vi "Activation Message Loop.vi"(8 "error in (no error)":errorcluster) -> (0 "error out":errorcluster)   [LabVIEW 2020, in "OPC.lvlib"]
doc: "Message loop for handling messages pertaining to the acquisition of data from the hardware."
uses:
  OPC.lvlib
  support/PCT FGV CMD.ctl
  Acquisition State.ctl
  AM Configuration.ctl
  support/Message Queue/Message Cluster.ctl
  support/Message Queue/Enqueue Message (Single).vi
  support/Message Queue/Message Queue.lvlib
  <vilib>/ErrorRing/Error Ring.xnode
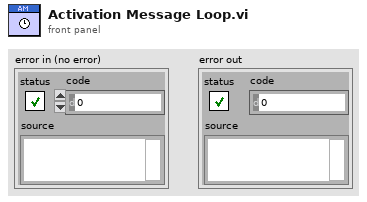
[diagram p1: front panel]
types:
  T1 = typedef "PCT FGV CMD.ctl" = enum16{"INIT", "GET", "SET"}
  T2 = typedef "PCT Data REFs.ctl" = cluster{"PLC AI Notifier":refnum<notifier>, "PS Data Queue":refnum<queue>, "BTN Queue":refnum<queue>, "PLC DI notifier":refnum<notifier>, "Timer notifier":refnum<notifier>, "DMM PS":refnum<notifier>, "DMM Gages":refnum<notifier>, "XYZ notifier":refnum<notifier>, "Test Notifier":refnum<notifier>, "Scanner notifier":refnum<notifier>, "OPC Notifier":refnum<notifier>, "HIDEN queue":refnum<queue>}
  T3 = typedef "Message Queue.lvlib/All Message Queues.ctl" = cluster{"UI":refnum<queue>, "Logging":refnum<queue>, "LOG":refnum<queue>, "ALARM":refnum<queue>, "Test":refnum<queue>, "Answer":refnum<queue>, "PLC":refnum<queue>, "DB":refnum<queue>, "Report":refnum<queue>, "OPC":refnum<queue>, "Procedure":refnum<queue>, "PalmSens":refnum<queue>, "SYS 7000 Reader":refnum<queue>, "SWITCH":refnum<queue>, "MOTOR":refnum<queue>, "MOTION":refnum<queue>, "HIDEN":refnum<queue>, "VALVE":refnum<queue>, "MFC":refnum<queue>, "PUMP IN":refnum<queue>, "PUMP OUT":refnum<queue>}
  T4 = typedef "OPC.lvlib/AM Configuration.ctl" = cluster{"Wait":dbl, "Next Step":string, "Writer Queue":refnum<queue>, "Reset":bool}
  T5 = typedef "OPC.lvlib/Acquisition State.ctl" = enum16{"Idle", "Initialized"}
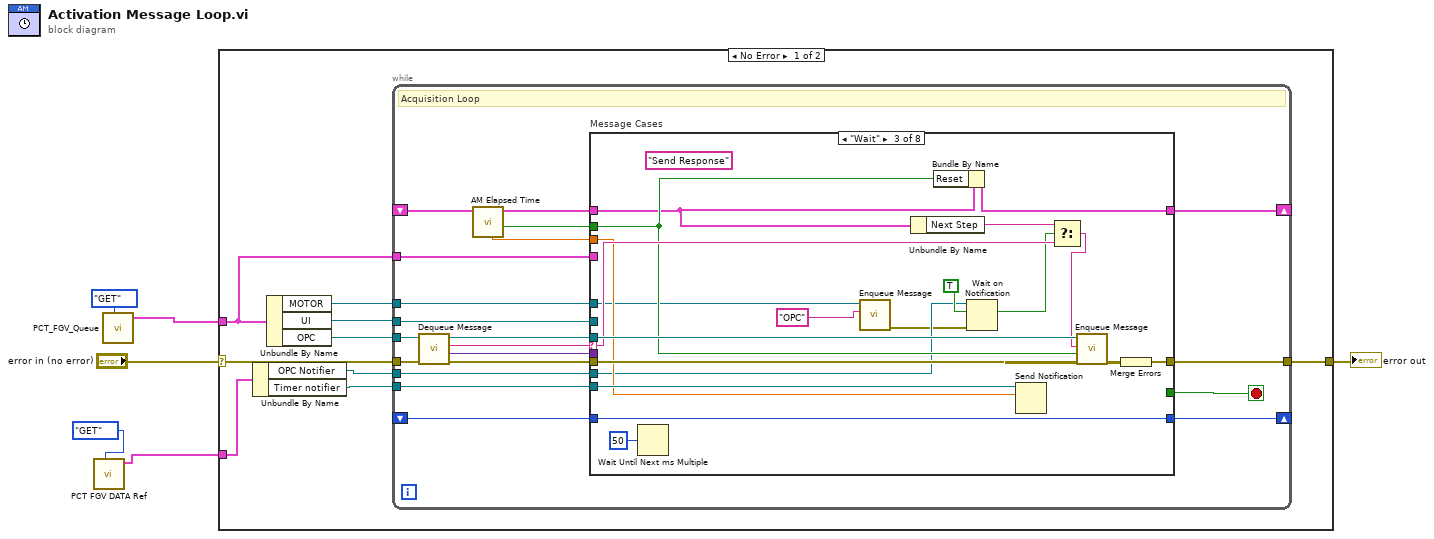
[diagram p0: block diagram]
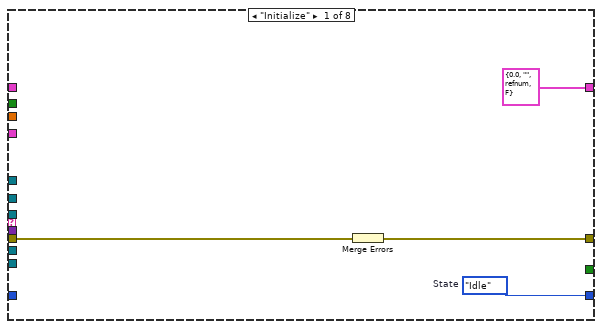
[diagram p2: hidden frame]
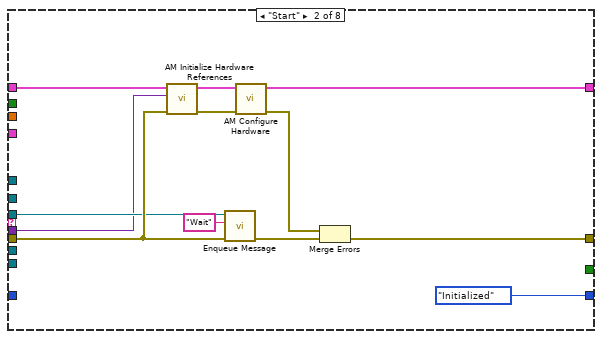
[diagram p3: hidden frame]
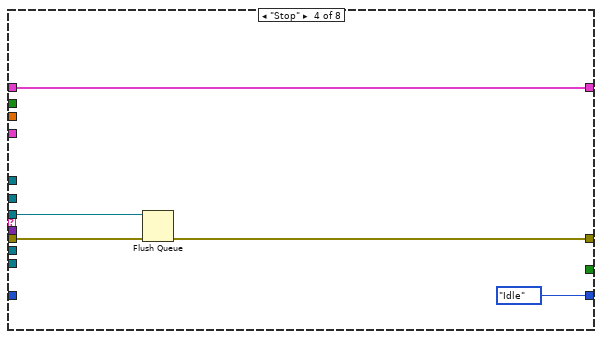
[diagram p4: hidden frame]
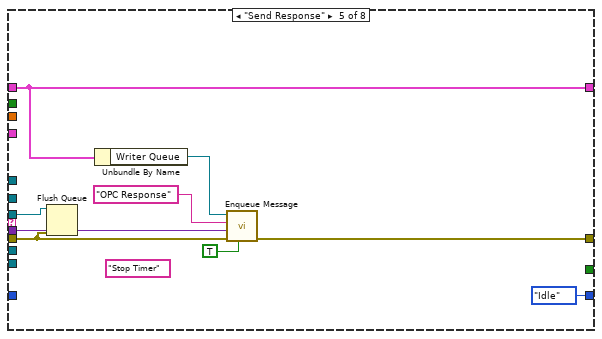
[diagram p5: hidden frame]
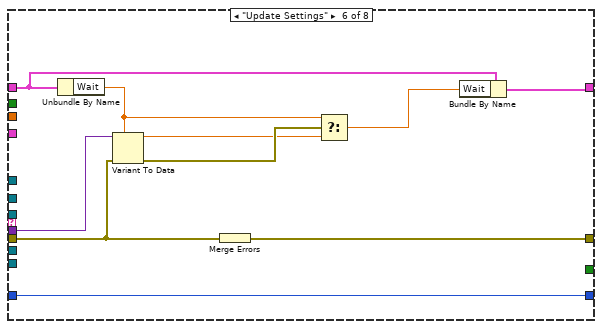
[diagram p6: hidden frame]
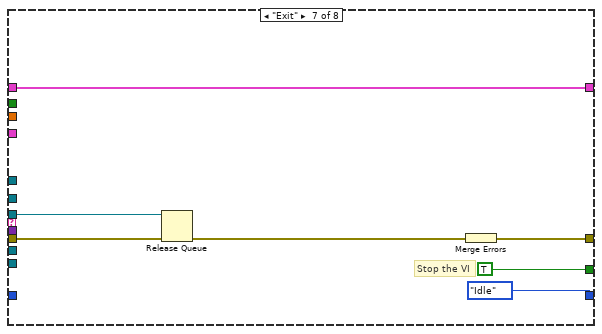
[diagram p7: hidden frame]
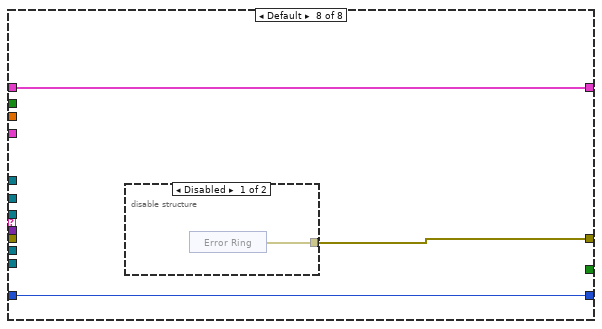
[diagram p8: hidden frame]
diagram:
  n1 = call "PCT FGV DATA Ref.vi"("CMD"=PCT_FGV_CMD."GET") -> ("Data REF"=w3:T2)  [unwired: 9 in, 1 out]
  n2 = call "PCT_FGV_Queue.vi"("CMD"=PCT_FGV_CMD."GET") -> ("Message Queues out"=w1:T3)  [unwired: 9 in, 1 out]
  n3 = case shown="No Error" "error in (no error)" {
    selector: "error in (no error)" -> [w13 w108]
    tunnel: w1 -> [w11 _]
    tunnel: [w14 w108] -> w6
    tunnel: w3 -> [w10 _]
    frame No Error {
      n4 = Unbundle By Name(w10) -> ("OPC Notifier"=w7:refnum<notifier>, "Timer notifier"=w9:refnum<notifier>)
      n5 = Unbundle By Name(w11) -> ("MOTOR"=w8:refnum<queue>, "UI"=w12:refnum<queue>, "OPC"=w15:refnum<queue>)
      n6 = while {
        tunnel: w15 -> [w29]
        shift-right: [w35] -> _
        shift-left: _ -> [w18]
        tunnel: w12 -> [w25]
        shift-right: [w27] -> _
        shift-left: _ -> [w28]
        tunnel: w11 -> [w21]
        tunnel: w13 -> [w33]
        tunnel: [w19] -> w14
        tunnel: w9 -> [w20]
        tunnel: w8 -> [w17]
        tunnel: w7 -> [w16]
        stop <- w34 stop-if-true
        # "Acquisition Loop"
        n7 = call "Dequeue Message.vi"("error in (no error)"=w33, "Message Queue"=w29) -> ("error out"=w32:errorcluster, "Message Data"=w30:variant, "Message"=w31:string, "dup Message Queue"=w26:refnum<queue>)  [unwired: 6 in]
        n8 = call "AM Elapsed Time.vi"("AM Refs in"=w18) -> ("Time has Elapsed"=w23:bool, "AM Refs out"=w24:T4, "Elapsed Time (s)"=w22:dbl)  [unwired: 8 in]
        n9 = case "Message Cases" shown="\"Wait\"" w31 {
          selector: w31 -> [_ _ w63 _ _ _ _ _]
          tunnel: w26 -> [_ w48 w67 w75 w79 _ w97 _]
          tunnel: w32 -> [w38 w49 w68 w73 w78 w91 w99 _]
          tunnel: [w39 w51 w70 w72 w85 w95 w101 w103] -> w19
          tunnel: w24 -> [_ w50 w59 w76 w83 w88 w100 w105]
          tunnel: [T4 {"Wait"=0.0, "Next Step"="", "Writer Queue"=refnum, "Reset"=FALSE} ("Data Cluster") w47 w64 w76 w83 w87 w100 w105] -> w35
          tunnel: [_ _ _ _ _ _ TRUE _] -> w34
          tunnel: w30 -> [_ w45 _ _ w84 w94 _ _]
          tunnel: w25 -> [_ _ _ _ _ _ _ _]
          tunnel: w28 -> [_ _ w71 _ _ w90 _ w104]
          tunnel: [w37 Acquisition_State."Initialized" ("Acquisition State") w71 Acquisition_State."Idle" ("Acquisition State") Acquisition_State."Idle" ("Acquisition State") w90 Acquisition_State."Idle" ("Acquisition State") w104] -> w27
          tunnel: w23 -> [_ _ w60 _ _ _ _ _]
          tunnel: w22 -> [_ _ w61 _ _ _ _ _]
          tunnel: w21 -> [_ _ _ _ _ _ _ _]
          tunnel: w20 -> [_ _ w62 _ _ _ _ _]
          tunnel: w17 -> [_ _ w54 _ _ _ _ _]
          tunnel: w16 -> [_ _ w56 _ _ _ _ _]
          frame "Initialize" {
            w37 = Acquisition_State."Idle"  # State
            # "Initialize  - Initialize is currently a no-op.  The hardware initialization takes place in the 'Start' message."
            n10 = Merge Errors(w38) -> (w39:errorcluster)
          }
          frame "Start" {
            # "Start - Configure and start the acquisition."
            n11 = call "AM Initialize Hardware References.vi"("error in (no error)"=w49, "Message Data"=w45, "Hardware Resources in"=w50) -> ("error out"=w44:errorcluster, "Hardware Resources out"=w42:T4)  [unwired: 7 in]
            n12 = call-poly "Enqueue Message.vi"("error in (no error)"=w49, "Message"="Wait", "Message Queue"=w48) -> ("error out"=w41:errorcluster)  [unwired: 7 in, 1 out]
            n13 = call "AM Configure Hardware.vi"("error in (no error)"=w44, "Hardware Resources in"=w42) -> ("error out"=w43:errorcluster, "Hardware Resources out"=w47:T4)  [unwired: 8 in]
            n14 = Merge Errors(w43, w41) -> (w51:errorcluster)
          }
          frame "Wait" {
            (unwired) "Send Response" ("Next Step")
            # "Start - Configure and start the acquisition."
            n15 = Wait Until Next ms Multiple(millisecond multiple=u32 50) -> ()  [unwired: 1 out]
            n16 = call-poly "Enqueue Message.vi"("Message"="OPC" ("Main CMD"), "Message Queue"=w54) -> ("error out"=w53:errorcluster)  [unwired: 8 in, 1 out]
            n17 = Unbundle By Name(w59) -> ("Next Step"=w58:string)
            n18 = Bundle By Name(cluster=w59, "Reset"=w60) -> (w64:T4)
            n19 = Wait on Notification(notifier=w56, ignore previous (F)=TRUE, error in (no error)=w53) -> (notification=w55:bool)  [unwired: 1 in, 3 out]
            n20 = Send Notification(notification=w61, notifier=w62) -> ()  [unwired: 1 in, 2 out]
            n21 = Select(t=w58, s=w55, f=w63) -> (s? t:f=w66:string)
            n22 = call-poly "Enqueue Message.vi"("error in (no error)"=w68, "Message Data"=w60, "Message"=w66, "Message Queue"=w67) -> ("error out"=w69:errorcluster)  [unwired: 6 in, 1 out]
            n23 = Merge Errors(w69) -> (w70:errorcluster)
          }
          frame "Stop" {
            # "Start - Configure and start the acquisition."
            n24 = Flush Queue(queue=w75, error in (no error)=w73) -> (error out=w72:errorcluster)  [unwired: 2 out]
          }
          frame "Send Response" {
            (unwired) "Stop Timer" ("Next Step")
            # "Acquire - Acquire data from the hardware. Since this is a continuous acquisition, this message will always message itself to run again."
            n25 = Flush Queue(queue=w79, error in (no error)=w78) -> ()  [unwired: 3 out]
            n26 = Unbundle By Name(w83) -> ("Writer Queue"=w82:refnum<queue>)
            n27 = call-poly "Enqueue Message.vi"("Priority Message? (F)"=TRUE, "error in (no error)"=w78, "Message Data"=w84, "Message"="OPC Response", "Message Queue"=w82) -> ("error out"=w85:errorcluster)  [unwired: 5 in, 1 out]
          }
          frame "Update Settings" {
            # "New settings are available, update the current ones stored in the shift register with the settings sent as part of the message"
            n28 = Unbundle By Name(w88) -> ("Wait"=w89:dbl)
            n29 = Variant To Data(error in=w91, type=w89, Variant=w94) -> (data=w92:dbl, error out=w93:errorcluster)
            n30 = Merge Errors(w91) -> (w95:errorcluster)
            n31 = Select(t=w89, s=w93, f=w92) -> (s? t:f=w86:dbl)
            n32 = Bundle By Name(cluster=w88, "Wait"=w86) -> (w87:T4)
          }
          frame "Exit" {
            # "Stop the VI"
            # "Exit - Send the Exit message to the UI Message Handler."
            n33 = Release Queue(queue=w97, error in (no error)=w99) -> (error out=w98:errorcluster)  [unwired: 1 in, 2 out]
            n34 = Merge Errors(w98) -> (w101:errorcluster)
          }
          frame Default {
            # "'Default' case only runs if there is a message that isn't defined in any of the other cases.  Output a programming error."
            n35 = disable-structure shown="Disabled" {
              disable-tunnel: [w106 _] -> w103
              frame Disabled {
                n36 = xnode "Error Ring"() -> ("error out"=w106:errorcluster)
              }
              frame Enabled {
              }
            }
          }
        }
      }
    }
    frame Error {
    }
  }
  "error out" <- w6
